vi "PLC Get Shift.vi"(6 "CID":string[](array[string]), 8 "error in (no error)":errorcluster, 9 "Current Time":timestamp, 10 "Time Stamp Out":timestamp[](array[timestamp]), 11 "connection reference in":T1) -> (0 "error out":errorcluster, 2 "Shift":i32, 3 "connection reference out":T1)   [LabVIEW 2017]
uses:
  <vilib>/addons/database/Connection.llb/Conn ObjectReference.ctl
  <userlib>/_OpenG.lib/comparison/comparison.llb/I32 Changed__ogtk.vi
  <vilib>/addons/database/Connection.llb/Conn Execute.vi
  <vilib>/addons/database/Recordset.llb/Rec Fetch Recordset Data (R).vi
  <vilib>/addons/database/Recordset.llb/Rec Destroy - Connection.vi
  <vilib>/addons/database/_DB Variant To Data/Database Variant To Data.xnode
  <vilib>/addons/database/NI_Database_API.lvlib
panel:
  out "double precision float":dbl format="%#_13g"
  in  "Shift Time Details":T2 {"3End" format="%<%H:%M:%S\n%x>T"; "2End" format="%<%H:%M:%S\n%x>T"; "3Start" format="%<%H:%M:%S\n%x>T"; "2Start" format="%<%H:%M:%S\n%x>T"; "1End" format="%<%H:%M:%S\n%x>T"; "1Start" format="%<%H:%M:%S\n%x>T"}
  # "Start Time"
  # "End Time"
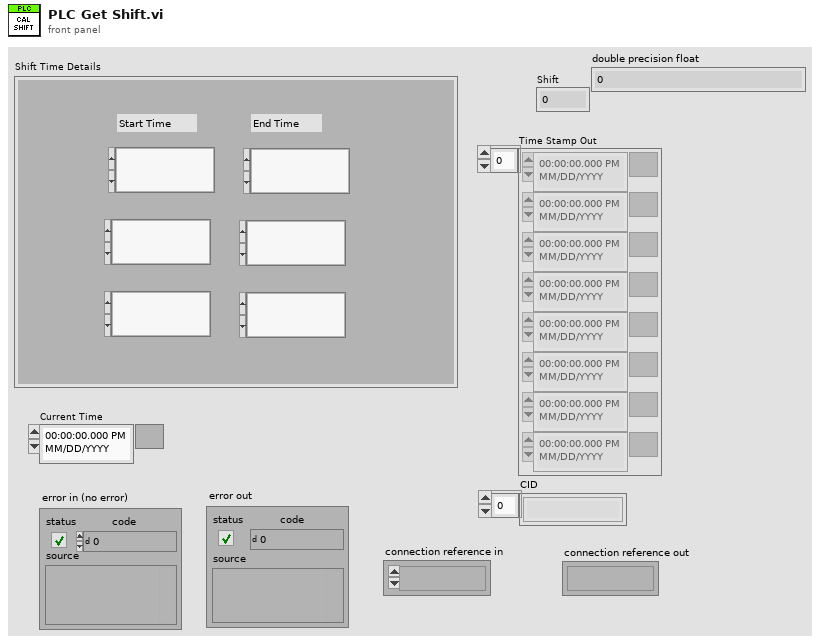
[diagram p1: front panel]
types:
  T1 = typedef "NI_Database_API.lvlib/Conn ObjectReference.ctl" = refnum<k1>
  T2 = cluster{"1Start":timestamp, "1End":timestamp, "2Start":timestamp, "3Start":timestamp, "2End":timestamp, "3End":timestamp}
  T3 = typedef "LVDateTimeRec.ctl" = cluster{"fractional second":dbl, "second":i32, "minute":i32, "hour":i32, "day of month":i32, "month":i32, "year":i32, "day of week":i32, "day of year":i32, "DST":i32}
  T4 = typedef "NI_Database_API.lvlib/Rec ObjectReference.ctl" = refnum<k1>
  T5 = cluster{i32, i32, i32, i32, "date/time string":string, "Date String":string}
  T6 = cluster{i32, "date/time string":string, i32, i32, i32, "Date String":string}
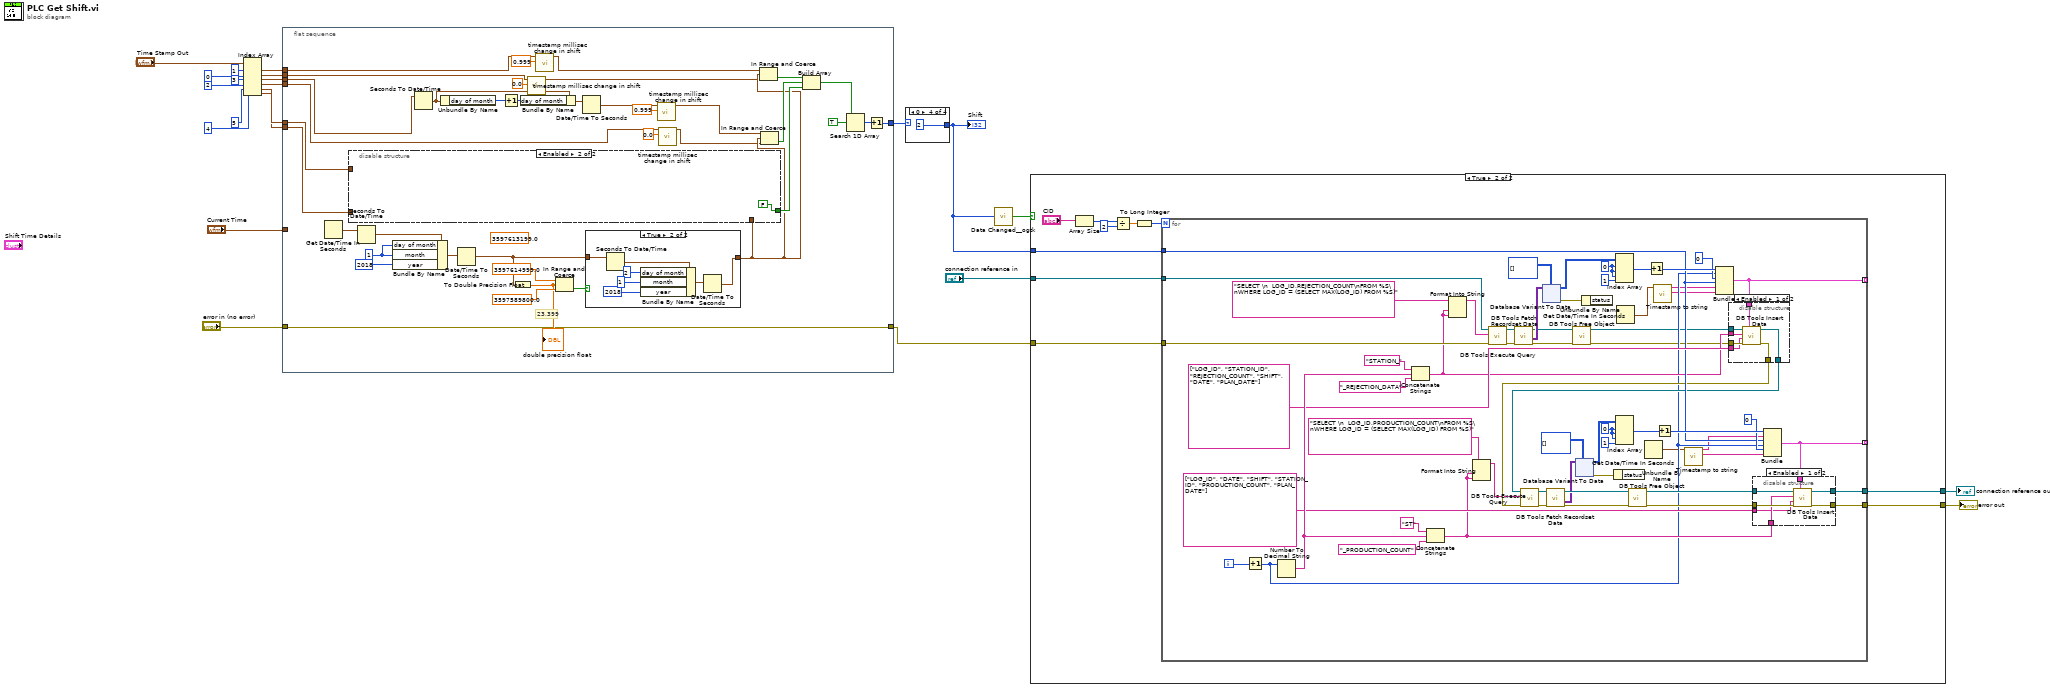
[diagram p0: block diagram]
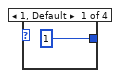
[diagram p5: hidden frame]
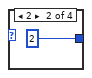
[diagram p6: hidden frame]
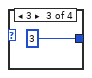
[diagram p7: hidden frame]
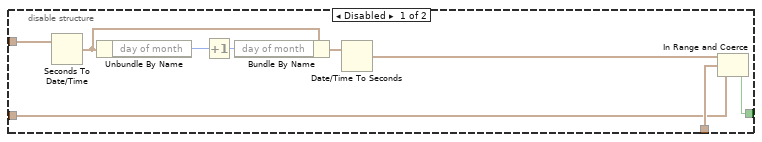
[diagram p8: hidden frame]
diagram:
  n1 = Index Array(array="Time Stamp Out", index #1=1 ("index"), index #2=0 ("index"), index #3=3 ("index"), index #4=2 ("index"), index #5=5 ("index"), index #6=4 ("index")) -> (element #1=w17:timestamp, element #2=w16:timestamp, element #3=w13:timestamp, element #4=w12:timestamp, element #5=w9:timestamp, element #6=w8:timestamp)
  n2 = flat-sequence {
    tunnel: [w54] -> w7
    tunnel: "error in (no error)" -> [w43]
    tunnel: [w43] -> w2
    tunnel: "Current Time" -> [_]
    tunnel: w17 -> [w34]
    tunnel: w16 -> [w30]
    tunnel: w13 -> [w35]
    tunnel: w12 -> [w25]
    tunnel: w9 -> [w42]
    tunnel: w8 -> [w41]
    frame #0 {
      (unwired) 3597613199.0 ("double precision float 2")
      w47 = 1 ("day of month")
      # "23,399"
      n3 = Get Date/Time In Seconds() -> (seconds since 1Jan1904=w40:timestamp)
      n4 = Seconds To Date/Time(time stamp (now)=w40) -> (date time rec=w51:T3)  [unwired: 1 in]
      n5 = Bundle By Name(cluster=w51, "day of month"=w47, "month"=w47, "year"=2018) -> (w53:T3)
      n6 = Seconds To Date/Time(time stamp (now)=w35) -> (date time rec=w38:T3)  [unwired: 1 in]
      n7 = Unbundle By Name(w38) -> ("day of month"=w36:i32)
      n8 = Date/Time To Seconds(2:w53) -> (0:w45:timestamp)  [unwired: 1 in]
      n9 = Increment(x=w36) -> (x+1=w37:i32)
      n10 = To Double Precision Float(number=w45) -> (double precision float=w48:dbl)
      "double precision float" <- w48
      n11 = Bundle By Name(cluster=w38, "day of month"=w37) -> (w39:T3)
      n12 = call "timestamp millisec change in shift.vi"("fractional second"=0.0, "time stamp in"=w30) -> ("time stamp out"=w29:timestamp)  [unwired: 9 in]
      n13 = call "timestamp millisec change in shift.vi"("fractional second"=0.999, "time stamp in"=w34) -> ("time stamp out"=w33:timestamp)  [unwired: 9 in]
      n14 = In Range and Coerce(upper limit=3597614999.0 ("double precision float 2"), x=w48, lower limit=3597589800.0 ("double precision float")) -> (In Range?=w46:bool)  [unwired: 1 out]
      n15 = Date/Time To Seconds(2:w39) -> (0:w28:timestamp)  [unwired: 1 in]
      n16 = case shown="True" w46 {
        tunnel: w45 -> [w71 w74]
        tunnel: [w71 w73] -> w44
        frame False {
        }
        frame True {
          n17 = Seconds To Date/Time(time stamp (now)=w74) -> (date time rec=w76:T3)  [unwired: 1 in]
          n18 = Bundle By Name(cluster=w76, "day of month"=2, "month"=1 ("day of month"), "year"=2018) -> (w78:T3)
          n19 = Date/Time To Seconds(2:w78) -> (0:w73:timestamp)  [unwired: 1 in]
        }
      }
      n20 = disable-structure shown="Enabled" {
        disable-tunnel: [w68 FALSE] -> w58
        disable-tunnel: w44 -> [w67 _]
        disable-tunnel: w42 -> [w66 _]
        disable-tunnel: w41 -> [w65 _]
        frame Disabled {
          n21 = Seconds To Date/Time(time stamp (now)=w66) -> (date time rec=w63:T3)  [unwired: 1 in]
          n22 = Unbundle By Name(w63) -> ("day of month"=w61:i32)
          n23 = Increment(x=w61) -> (x+1=w62:i32)
          n24 = Bundle By Name(cluster=w63, "day of month"=w62) -> (w64:T3)
          n25 = Date/Time To Seconds(2:w64) -> (0:w69:timestamp)  [unwired: 1 in]
          n26 = In Range and Coerce(upper limit=w69, x=w67, lower limit=w65) -> (In Range?=w68:bool)  [unwired: 1 out]
        }
        frame Enabled {
        }
      }
      n27 = call "timestamp millisec change in shift.vi"("fractional second"=0.999, "time stamp in"=w28) -> ("time stamp out"=w27:timestamp)  [unwired: 9 in]
      n28 = call "timestamp millisec change in shift.vi"("fractional second"=0.0, "time stamp in"=w25) -> ("time stamp out"=w24:timestamp)  [unwired: 9 in]
      n29 = In Range and Coerce(upper limit=w33, x=w44, lower limit=w29) -> (In Range?=w60:bool)  [unwired: 1 out]
      n30 = In Range and Coerce(upper limit=w27, x=w44, lower limit=w24) -> (In Range?=w59:bool)  [unwired: 1 out]
      n31 = Build Array(w60, w59, w58) -> (w57:bool[])
      n32 = Search 1D Array(1D array=w57, element=TRUE) -> (index of element=w55:i32)  [unwired: 1 in]
      n33 = Increment(x=w55) -> (x+1=w54:i32)
    }
  }
  n34 = case shown="0" w7 {
    tunnel: [1 2 3 2] -> w4
    frame 1, Default {
    }
    frame 2 {
    }
    frame 3 {
    }
    frame 0 {
    }
  }
  "Shift" <- w4
  n35 = call-poly <userlib>:"Data Changed__ogtk.vi"("I32"=w4) -> ("Changed"=w1:bool)
  n36 = case shown="True" w1 {
    tunnel: [w84 w90] -> w6
    tunnel: "connection reference in" -> [w84 w89]
    tunnel: w4 -> [_ w88]
    tunnel: [w83 w87] -> w3
    tunnel: w2 -> [w83 w86]
    frame False {
    }
    frame True {
      n37 = Array Size(array="CID") -> (size(s)=w93:i32)
      n38 = Divide(x=w93, y=2) -> (x/y=w91:dbl)
      n39 = To Long Integer(number=w91) -> (32bit integer=w85:i32)
      n40 = for {
        N: w85 -> [_]
        tunnel: [w136] -> w87
        tunnel: [w135] -> w90
        tunnel: w89 -> [w129]
        tunnel: w88 -> [w134]
        tunnel: w86 -> [w128]
        tunnel: [w107] -> _ mode=indexing
        tunnel: [w106] -> _ mode=indexing
        i -> [w143]
        w146 = 0 ("index (row)")
        w149 = 0 ("index (row)")
        n41 = Increment(x=w143) -> (x+1=w105:i32)
        n42 = Number To Decimal String(number=w105) -> (decimal integer string=w142:string)  [unwired: 1 in]
        n43 = Concatenate Strings("STATION_" ("String"), w142, "_REJECTION_DATA" ("string")) -> (w123:string)
        n44 = Concatenate Strings("ST" ("String"), w142, "_PRODUCTION_COUNT" ("string")) -> (w108:string)
        n45 = Format Into String(format string="SELECT \n  LOG_ID,REJECTION_COUNT\nFROM %S\nWHERE LOG_ID = (SELECT MAX(LOG_ID) FROM %S)" ("SQL query"), w123, w123) -> (resulting string=w126:string)  [unwired: 2 in, 1 out]
        n46 = Format Into String(format string="SELECT \n  LOG_ID,PRODUCTION_COUNT\nFROM %S\nWHERE LOG_ID = (SELECT MAX(LOG_ID) FROM %S)" ("SQL query"), w108, w108) -> (resulting string=w109:string)  [unwired: 2 in, 1 out]
        n47 = call-poly <vilib>:"DB Tools Execute Query.vi"("error in (no error)"=w128, "SQL query"=w126, "connection reference"=w129) -> ("error out"=w133:errorcluster, "recordset reference"=w103:T4)  [unwired: 5 in]
        n48 = call-poly <vilib>:"DB Tools Fetch Recordset Data.vi"("error in (no error)"=w133, "recordset reference"=w103) -> ("error out"=w130:errorcluster, "recordset data"=w132:variant[][], "recordset reference out"=w104:T4)  [unwired: 3 in]
        n49 = xnode "Database Variant To Data"("database variant"=w132, "type"=i32[][] []) -> ("data"=w125:i32[][], "error out"=w124:errorcluster)  [unwired: 1 in]
        n50 = call-poly <vilib>:"DB Tools Free Object.vi"("error in (no error)"=w130, "recordset reference"=w104) -> ("error out"=w102:errorcluster, "connection reference"=w101:T1)  [unwired: 8 in]
        n51 = Unbundle By Name(w124) -> ()  [unwired: 1 out]
        n52 = Index Array(array=w125, index (row) #1=w149, index (col) #1=w149, index (row) #2=w149, index (col) #2=1 ("disabled index (col)")) -> (element #1=w153:i32)  [unwired: 1 out]
        n53 = Get Date/Time In Seconds() -> (seconds since 1Jan1904=w100:timestamp)
        n54 = Get Date/Time In Seconds() -> (seconds since 1Jan1904=w99:timestamp)
        n55 = Increment(x=w153) -> (x+1=w154:i32)
        n56 = call "Timestamp to string.vi"("time stamp"=w100) -> ("Date String"=w95:string, "date/time string"=w96:string)  [unwired: 8 in, 1 out]
        n57 = call "Timestamp to string.vi"("time stamp"=w99) -> ("Date String"=w97:string, "date/time string"=w98:string)  [unwired: 8 in, 1 out]
        n58 = Bundle(w154, w105, 0, w134, "date/time string"=w96, "Date String"=w95) -> (w106:T5)  [unwired: 1 in]
        n59 = disable-structure shown="Enabled" {
          disable-tunnel: w123 -> [w258 _]
          disable-tunnel: w101 -> [w257 w260]
          disable-tunnel: w102 -> [w256 w259]
          disable-tunnel: w106 -> [w255 _]
          disable-tunnel: string[] ["LOG_ID", "STATION_ID", "REJECTION_COUNT", "SHIFT", "DATE", "PLAN_DATE"] ("columns") -> [w254 _]
          disable-tunnel: [w253 w260] -> w116
          disable-tunnel: [w252 w259] -> w115
          frame Enabled {
            n60 = call <vilib>:"DB Tools Insert Data.vi"("data"=w255, "error in (no error)"=w256, "columns"=w254, "table"=w258, "connection reference"=w257) -> ("error out"=w252:errorcluster, "connection reference out"=w253:T1)  [unwired: 5 in]
          }
          frame Disabled {
          }
        }
        n61 = call-poly <vilib>:"DB Tools Execute Query.vi"("error in (no error)"=w115, "SQL query"=w109, "connection reference"=w116) -> ("error out"=w120:errorcluster, "recordset reference"=w119:T4)  [unwired: 5 in]
        n62 = call-poly <vilib>:"DB Tools Fetch Recordset Data.vi"("error in (no error)"=w120, "recordset reference"=w119) -> ("error out"=w122:errorcluster, "recordset data"=w111:variant[][], "recordset reference out"=w121:T4)  [unwired: 3 in]
        n63 = xnode "Database Variant To Data"("database variant"=w111, "type"=i32[][] []) -> ("data"=w112:i32[][], "error out"=w114:errorcluster)  [unwired: 1 in]
        n64 = Unbundle By Name(w114) -> ()  [unwired: 1 out]
        n65 = Index Array(array=w112, index (row) #1=w146, index (col) #1=w146, index (row) #2=w146, index (col) #2=1 ("disabled index (col)")) -> (element #1=w137:i32)  [unwired: 1 out]
        n66 = call-poly <vilib>:"DB Tools Free Object.vi"("error in (no error)"=w122, "recordset reference"=w121) -> ("error out"=w118:errorcluster, "connection reference"=w117:T1)  [unwired: 8 in]
        n67 = Increment(x=w137) -> (x+1=w139:i32)
        n68 = Bundle(w139, "date/time string"=w98, w134, w105, 0, "Date String"=w97) -> (w107:T6)  [unwired: 1 in]
        n69 = disable-structure shown="Enabled" {
          disable-tunnel: w118 -> [w249 w250]
          disable-tunnel: w117 -> [w248 w251]
          disable-tunnel: w108 -> [w247 _]
          disable-tunnel: string[] ["LOG_ID", "DATE", "SHIFT", "STATION_ID", "PRODUCTION_COUNT", "PLAN_DATE"] ("columns") -> [w246 _]
          disable-tunnel: w107 -> [w245 _]
          disable-tunnel: [w244 w250] -> w136
          disable-tunnel: [w243 w251] -> w135
          frame Enabled {
            n70 = call <vilib>:"DB Tools Insert Data.vi"("data"=w245, "error in (no error)"=w249, "columns"=w246, "table"=w247, "connection reference"=w248) -> ("error out"=w244:errorcluster, "connection reference out"=w243:T1)  [unwired: 5 in]
          }
          frame Disabled {
          }
        }
      }
    }
  }
  "error out" <- w3
  "connection reference out" <- w6
